vi "Auto_Routine_Deposit_Balance.vi"(8 "error in (no error)":errorcluster) -> (0 "error out":errorcluster)   [LabVIEW 2020]
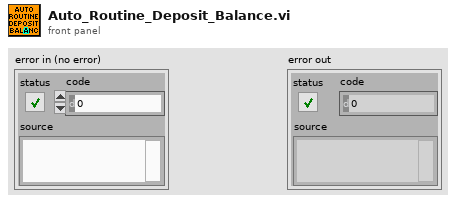
[diagram p1: front panel]
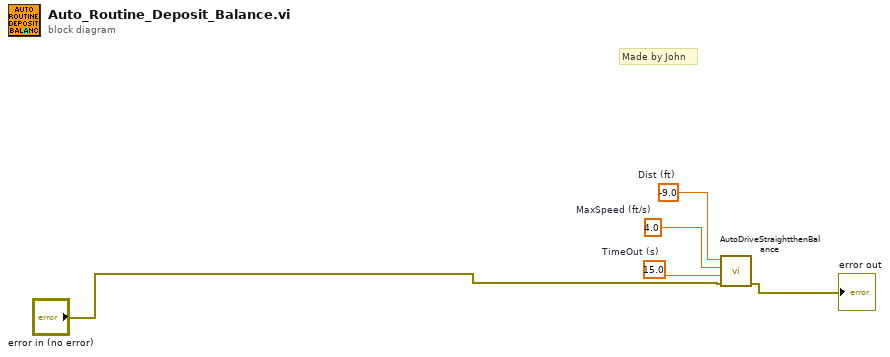
[diagram p0: block diagram]
diagram:
  w3 = 15.0  # TimeOut (s)
  w4 = 4.0  # MaxSpeed (ft/s)
  w5 = -9.0  # Dist (ft)
  # "Made by John"
  n1 = call "AutoDriveStraightthenBalance.vi"("error in (no error)"="error in (no error)", "TimeOut (s)"=w3, "MaxSpeed (ft/s)"=w4, "Dist (ft)"=w5) -> ("error out"=→"error out":errorcluster)  [unwired: 7 in]
